vi "Error Word Bits Checker for All Parameters on Label.vi"(6 "error text in":string, 8 "error in":errorcluster, 11 "parameters in":T1[](array[typedef])) -> (0 "error out":errorcluster, 3 "parameters out":T1[](array[typedef]))   [LabVIEW 2023]
uses:
  <vilib>/NI/NI VeriStand Encoding and Decoding/Encoding.ctl
  Parameter Definition.ctl
  VS Channel Definition for Parameter.ctl
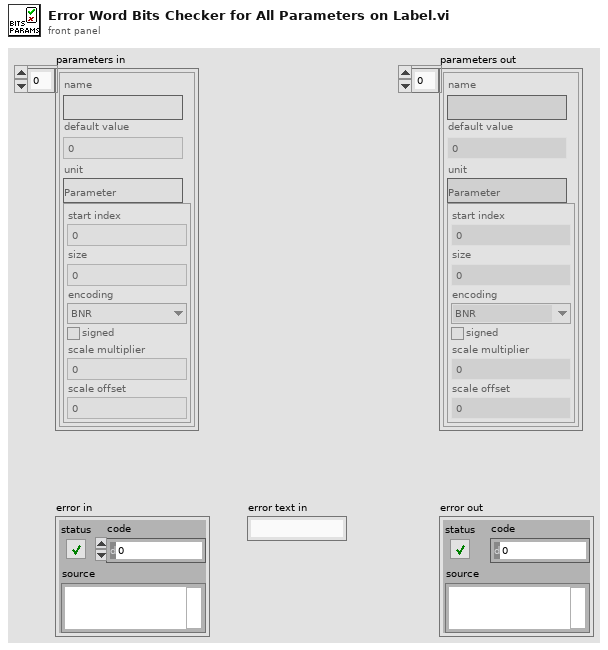
[diagram p1: front panel]
types:
  T1 = typedef "VS Channel Definition for Parameter.ctl" = cluster{"name":string, "default value":dbl, "unit":string, "Parameter":T2}
  T2 = typedef "Parameter Definition.ctl" = cluster{"start index":i32, "size":i32, "encoding":T3, "signed":bool, "scale multiplier":dbl, "scale offset":dbl}
  T3 = typedef "Encoding and Decoding.lvlib/Encoding.ctl" = enum16{"BNR", "BCD", "Discrete"}
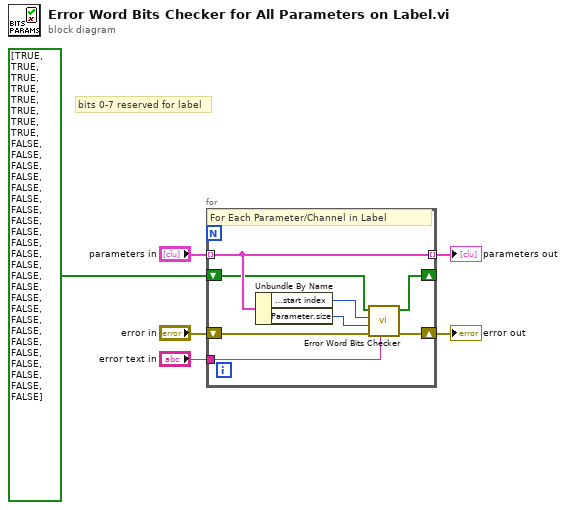
[diagram p0: block diagram]
diagram:
  # "bits 0-7 reserved for label"
  n1 = for {
    shift-right: [w13] -> w3
    shift-left: "error in" -> [w14]
    tunnel: "parameters in" -> [w11] mode=indexing
    tunnel: "error text in" -> [w12]
    tunnel: [w11] -> w6 mode=indexing
    shift-right: [w7] -> _
    shift-left: bool[] [TRUE, TRUE, TRUE, TRUE, TRUE, TRUE, TRUE, TRUE, FALSE, FALSE, FALSE, FALSE, FALSE, FALSE, FALSE, FALSE, FALSE, FALSE, FALSE, FALSE, FALSE, FALSE, FALSE, FALSE, FALSE, FALSE, FALSE, FALSE, FALSE, FALSE, FALSE, FALSE] -> [w8]
    # "For Each Parameter/Channel in Label"
    n2 = Unbundle By Name(w11) -> ("Parameter.start index"=w10:i32, "Parameter.size"=w9:i32)
    n3 = call "Error Word Bits Checker.vi"("error text in"=w12, "error in"=w14, "number of bits"=w9, "start bit"=w10, "reserved bits in"=w8) -> ("error out"=w13:errorcluster, "reserved bits out"=w7:bool[])  [unwired: 5 in]
  }
  "parameters out" <- w6
  "error out" <- w3
